vi "PH_Sixpack_Switch.ProcCases.vi"(0 "i ref in":refnum<vi>, 1 "selector":string, 2 "Data":T1, 3 "call cluster":T2={"Object"="", "Selector"="", "CallType"=enum."synchronous", "Async Object"="", "Async Selector"="", "Data Descriptor"="", "Data"=[], "Error #"=0, "Expire"=0}, 5 "error in (no error)":errorcluster) -> (14 "i ref out":refnum<vi>, 17 "answer cluster":T2={"Object"="", "Selector"="", "CallType"=enum."synchronous", "Async Object"="", "Async Selector"="", "Data Descriptor"="", "Data"=[], "Error #"=0, "Expire"=0}, 19 "error out":errorcluster)   [LabVIEW 2014, in "PH_Sixpack_Switch.lvlib"]
doc: "This method is called by a process from within the default case in the event loop. The methods of a class that are linked to events will be called from THIS method. Add your code here."
uses:
  PH_Sixpack_Switch.lvlib
  CS_Core/CSSystem/CoreDefs/CoreDefs.call_type.ctl
  CS_Core/BaseProcess/BaseProcess.descriptor string definition.ctl
  CS_Core/CSSystem/CoreDefs/CoreDefs.rawDataType.ctl
  CS_Core/CSSystem/CoreLib/CoreLib.string 2 byte array.vi
  CS_Core/CSSystem/CoreLib/CoreLib.byte array 2 short.vi
  CS_Core/CSSystem/CoreLib/CoreLib.lvlib
  CS_Core/BaseProcess/BaseProcess.lvlib
  CS_Core/CAEObj/CAEObj.lvlib
  PH_Basics/PH_PSDBWriter/PH_PSDBWriter.lvlib
  PH_Basics/PH_AxisGUI_BaseClass/PH_AxisGUI_BaseClass.lvlib
  PH_Basics/PH_Stepmotor_BaseClass/PH_Stepmotor_BaseClass.lvlib
  PH_AxisGUI_6P/PH_AxisGUI_6P.lvlib
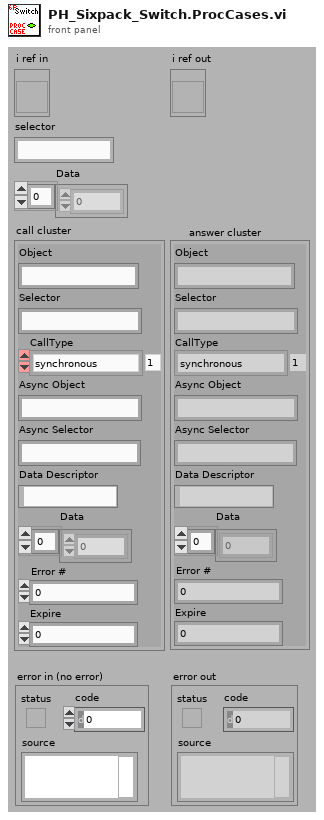
[diagram p1: front panel]
types:
  T1 = typedef "CoreDefs.rawDataType.ctl" = i8[]
  T2 = typedef "CoreDefs.call_type.ctl" = cluster{"Object":string, "Selector":string, "CallType":enum16{"simple", "synchronous", "asynchronous"}, "Async Object":string, "Async Selector":string, "Data Descriptor":T3, "Data":T1, "Error #":i32, "Expire":u32}
  T3 = typedef "BaseProcess.lvlib/BaseProcess.descriptor string definition.ctl" = string
  T4 = enum8{"Enabled", "Disabled", "Disabled and Grayed Out"}
  T5 = typedef "PH_Sixpack_Switch.lvlib/PH_Sixpack_Switch.i attribute.ctl" = cluster{"GUI Refs":cluster{"Delete":refnum<vi>, "Move":refnum<vi>, "Direction":refnum<vi>}, "remote controlled?":bool, "Move":bool, "Direction":T6}
  T6 = typedef "PH_Stepmotor_BaseClass.lvlib/PH_Stepmotor_BaseClass.Axis Direction.ctl" = enum16{"forward", "backward"}
  T7 = typedef "PH_Stepmotor_BaseClass.lvlib/PH_Stepmotor_BaseClass.Axis Information.ctl" = cluster{"Scaled Position":dbl, "Activity":T8}
  T8 = typedef "PH_Stepmotor_BaseClass.lvlib/PH_Stepmotor_BaseClass.Axis Activity.ctl" = enum16{"No Information", "stopped", "running", "Failure", "Alarm", "stopped at backward ES", "stopped at foreward ES"}
  T9 = typedef "PH_AxisGUI_BaseClass.lvlib/PH_AxisGUI_BaseClass.i attribute.ctl" = cluster{"Axes":T10[]}
  T10 = typedef "PH_AxisGUI_BaseClass.lvlib/PH_AxisGUI_BaseClass.Axis Attributes.ctl" = cluster{"Axis GUI Refs":T11, "Address":T12, "Name":string, "Label \"Back\"":string, "Labell \"Forth\"":string, "Moving?":bool}
  T11 = typedef "PH_AxisGUI_BaseClass.lvlib/PH_AxisGUI_BaseClass.Axis GUI Refs.ctl" = cluster{"Back":refnum<vi>, "Forth":refnum<vi>, "Status":refnum<vi>, "Target":refnum<vi>, "Address":refnum<vi>, "Status Bar":refnum<vi>, "Settings":refnum<vi>, "Activity":refnum<vi>, "Clear Error":refnum<vi>}
  T12 = typedef "PH_Stepmotor_BaseClass.lvlib/PH_Stepmotor_BaseClass.Axis Address.ctl" = cluster{"Instance":string, "Motor Nr":i32}
  T13 = typedef "PH_PSDBWriter.lvlib/PH_PSDBWriter.PHELIX-Subsystems.ctl" = i32
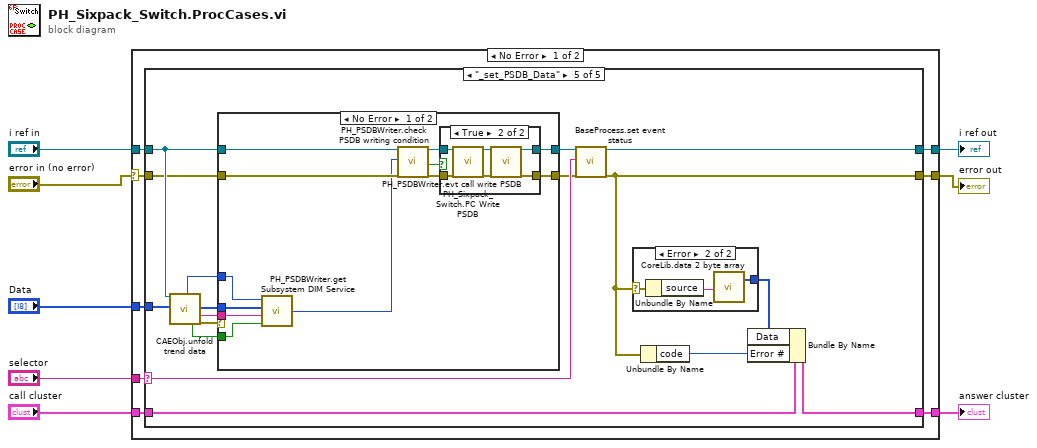
[diagram p0: block diagram]
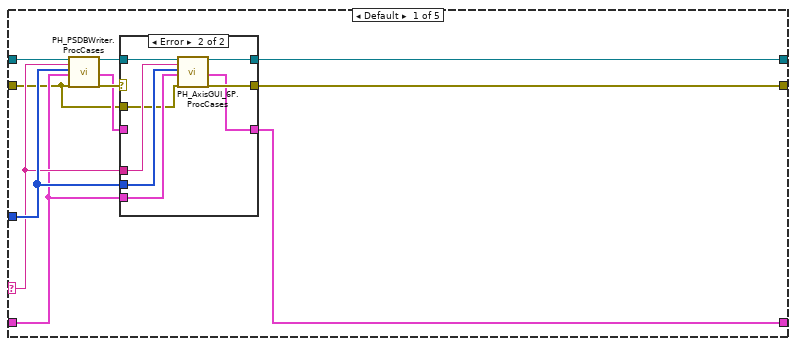
[diagram p2: hidden frame]
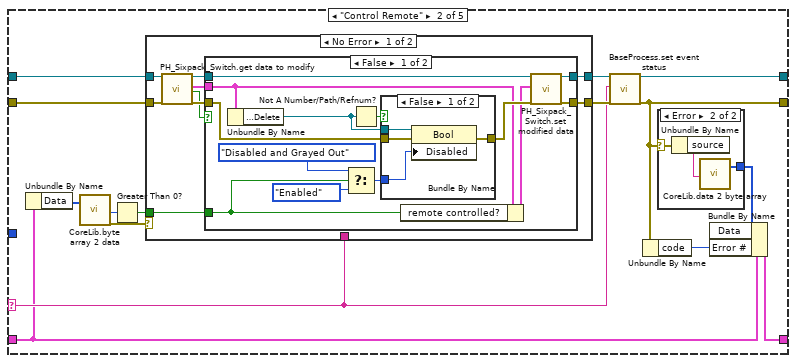
[diagram p4: hidden frame]
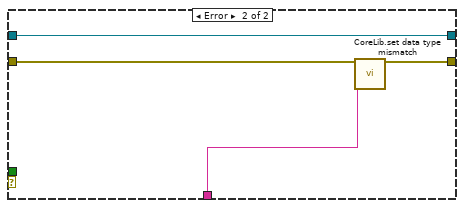
[diagram p8: hidden frame]
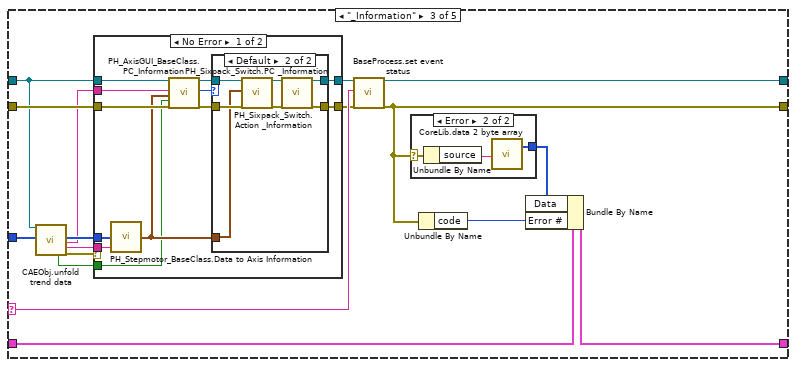
[diagram p9: hidden frame]
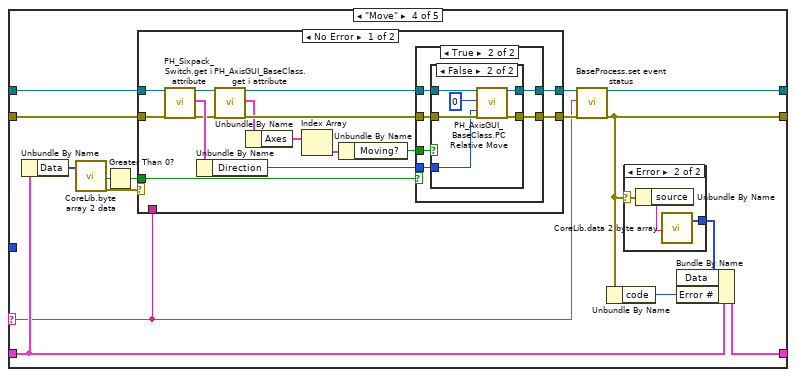
[diagram p13: hidden frame]
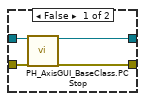
[diagram p14: hidden frame]
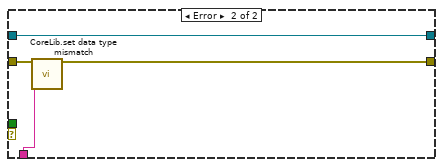
[diagram p16: hidden frame]
diagram:
  n1 = case shown="No Error" "error in (no error)" {
    selector: "error in (no error)" -> [w9 w231]
    tunnel: "selector" -> [w16 _]
    tunnel: [w15 w230] -> w7
    tunnel: "call cluster" -> [w14 w230]
    tunnel: "i ref in" -> [w13 w232]
    tunnel: [w12 w232] -> w4
    tunnel: [w11 w231] -> w3
    tunnel: "Data" -> [w10 _]
    frame No Error {
      n2 = case shown="\"_set_PSDB_Data\"" w16 {
        selector: w16 -> [w19 w41 w102 w134 w198]
        tunnel: w13 -> [w26 w45 w91 w139 w192]
        tunnel: [w25 w43 w104 w145 w202] -> w12
        tunnel: w14 -> [w18 w40 w101 w137 w199]
        tunnel: [w21 w39 w100 w143 w200] -> w15
        tunnel: w9 -> [w17 w44 w94 w141 w191]
        tunnel: [w24 w42 w103 w144 w201] -> w11
        tunnel: w10 -> [w20 _ w99 _ w190]
        frame Default {
          n3 = call "PH_PSDBWriter.ProcCases.vi"("i ref in"=w26, "selector"=w19, "Data"=w20, "call cluster"=w18, "error in"=w17) -> ("i ref out"=w27:refnum<vi>, "answer cluster"=w22:T2, "error out"=w23:errorcluster)  [unwired: 12 in]
          n4 = case shown="Error" w23 {
            selector: w23 -> [w29 _]
            tunnel: w27 -> [w30 w38]
            tunnel: [w30 w37] -> w25
            tunnel: [w29 w36] -> w24
            tunnel: w22 -> [w28 _]
            tunnel: [w28 w35] -> w21
            tunnel: w20 -> [_ w34]
            tunnel: w19 -> [_ w33]
            tunnel: w18 -> [_ w32]
            tunnel: w17 -> [_ w31]
            frame No Error {
            }
            frame Error {
              n5 = call "PH_AxisGUI_6P.ProcCases.vi"("i ref in"=w38, "selector"=w33, "data"=w34, "call cluster"=w32, "error in"=w31) -> ("i ref out"=w37:refnum<vi>, "answer cluster"=w35:T2, "error out"=w36:errorcluster)  [unwired: 12 in]
            }
          }
        }
        frame "Control Remote" {
          n6 = Unbundle By Name(w40) -> ("Data"=w48:T1)
          n7 = call-poly "CoreLib.byte array 2 data.vi"("byteArray"=w48) -> ("i16"=w49:i16, "error out"=w51:errorcluster)  [unwired: 16 in, 1 out]
          n8 = Greater Than 0?(x=w49) -> (x > 0?=w50:bool)
          n9 = case shown="No Error" w51 {
            tunnel: [w58 w89] -> w46
            tunnel: w45 -> [w65 w89]
            tunnel: w44 -> [w64 w88]
            tunnel: [w60 w87] -> w47
            tunnel: w41 -> [_ w86]
            tunnel: w50 -> [w62 _]
            frame No Error {
              n10 = call "PH_Sixpack_Switch.get data to modify.vi"("i ref in"=w65, "error in (no error)"=w64) -> ("i ref out"=w59:refnum<vi>, "i attribute"=w63:T5, "timed out"=w57:bool, "error out"=w61:errorcluster)  [unwired: 14 in]
              n11 = case shown="False" w57 {
                tunnel: w63 -> [w73 _]
                tunnel: w62 -> [w71 _]
                tunnel: w61 -> [w78 w84]
                tunnel: [w77 w84] -> w60
                tunnel: w59 -> [w75 w85]
                tunnel: [w74 w85] -> w58
                frame False {
                  n12 = Unbundle By Name(w73) -> ("GUI Refs.Delete"=w69:refnum<vi>)
                  n13 = Select(t=T4."Disabled and Grayed Out", s=w71, f=T4."Enabled" ("Disabled")) -> (s? t:f=w70:T4)
                  n14 = Not A Number/Path/Refnum?(number/path/refnum=w69) -> (NaN/Path/Refnum?=w68:bool)
                  n15 = case shown="False" w68 {
                    tunnel: w69 -> [w82 _]
                    tunnel: w78 -> [w81 w83]
                    tunnel: [w80 w83] -> w76
                    tunnel: w70 -> [w79 _]
                    frame False {
                      n16 = property class="Bool"(reference=w82, error in=w81, "Disabled"=w79) -> (error out=w80:errorcluster)  [unwired: 1 out]
                    }
                    frame True {
                    }
                  }
                  n17 = Bundle By Name(cluster=w73, "remote controlled?"=w71) -> (w72:T5)
                  n18 = call "PH_Sixpack_Switch.set modified data.vi"("i ref in"=w75, "i attribute"=w72, "error in (no error)"=w76) -> ("i ref out"=w74:refnum<vi>, "error out"=w77:errorcluster)  [unwired: 15 in]
                }
                frame True {
                }
              }
            }
            frame Error {
              n19 = call "CoreLib.set data type mismatch.vi"("error in (no error)"=w88, "error source"=w86) -> ("error out"=w87:errorcluster)  [unwired: 17 in]
            }
          }
          n20 = call "BaseProcess.set event status.vi"("i ref in"=w46, "EventStatus"=w41, "error in (no error)"=w47) -> ("i ref out"=w43:refnum<vi>, "error out"=w42:errorcluster)  [unwired: 14 in, 1 out]
          n21 = Unbundle By Name(w42) -> ("code"=w52:i32)
          n22 = case shown="Error" w42 {
            selector: w42 -> [_ w56]
            tunnel: [_ w54] -> w53
            frame No Error {
            }
            frame Error {
              n23 = Unbundle By Name(w56) -> ("source"=w55:string)
              n24 = call-poly "CoreLib.data 2 byte array.vi"("string"=w55) -> ("byteArray out"=w54:T1)  [unwired: 18 in]
            }
          }
          n25 = Bundle By Name(cluster=w40, "Data"=w53, "Error #"=w52) -> (w39:T2)
        }
        frame "_Information" {
          n26 = call "CAEObj.unfold trend data.vi"("i ref in"=w91, "raw trend data"=w99) -> ("no link"=w92:bool, "data"=w98:i8[], "serviceName"=w90:string, "typeDescriptor"=w97:string, "error out"=w96:errorcluster)  [unwired: 9 in, 4 out]
          n27 = case shown="No Error" w96 {
            tunnel: w98 -> [w111 _]
            tunnel: w97 -> [w110 _]
            tunnel: w91 -> [w114 w129]
            tunnel: [w117 w129] -> w95
            tunnel: w94 -> [w118 w128]
            tunnel: [w116 w128] -> w93
            tunnel: w92 -> [w107 _]
            tunnel: w90 -> [w112 _]
            frame No Error {
              n28 = call "PH_Stepmotor_BaseClass.Data to Axis Information.vi"("data"=w111, "Type Descriptor"=w110) -> ("Axis Information"=w108:T7)
              n29 = call "PH_AxisGUI_BaseClass.PC_Information.vi"("i ref in"=w114, "Service Name"=w112, "Axis Information"=w108, "no link"=w107, "error in"=w118) -> ("i ref out"=w113:refnum<vi>, "Axis"=w109:i32, "error out"=w115:errorcluster)  [unwired: 12 in]
              n30 = case shown="Default" w109 {
                tunnel: [w120 w122] -> w117
                tunnel: [w119 w121] -> w116
                tunnel: w115 -> [w119 w125]
                tunnel: w113 -> [w120 w124]
                tunnel: w108 -> [_ w123]
                frame -1 {
                }
                frame Default {
                  n31 = call "PH_Sixpack_Switch.PC _Information.vi"("i ref in"=w124, "Axis Information"=w123, "error IO"=w125) -> ("i ref out"=w127:refnum<vi>, "error out"=w126:errorcluster)  [unwired: 15 in]
                  n32 = call "PH_Sixpack_Switch.Action _Information.vi"("i ref in"=w127, "error IO"=w126) -> ("i ref out"=w122:refnum<vi>, "error out"=w121:errorcluster)  [unwired: 16 in]
                }
              }
            }
            frame Error {
            }
          }
          n33 = call "BaseProcess.set event status.vi"("i ref in"=w95, "EventStatus"=w102, "error in (no error)"=w93) -> ("i ref out"=w104:refnum<vi>, "error out"=w103:errorcluster)  [unwired: 14 in, 1 out]
          n34 = case shown="Error" w103 {
            selector: w103 -> [_ w132]
            tunnel: [_ w130] -> w106
            frame No Error {
            }
            frame Error {
              n35 = Unbundle By Name(w132) -> ("source"=w131:string)
              n36 = call-poly "CoreLib.data 2 byte array.vi"("string"=w131) -> ("byteArray out"=w130:T1)  [unwired: 18 in]
            }
          }
          n37 = Unbundle By Name(w103) -> ("code"=w105:i32)
          n38 = Bundle By Name(cluster=w101, "Data"=w106, "Error #"=w105) -> (w100:T2)
        }
        frame "Move" {
          n39 = Unbundle By Name(w137) -> ("Data"=w138:T1)
          n40 = call-poly "CoreLib.byte array 2 data.vi"("byteArray"=w138) -> ("i16"=w135:i16, "error out"=w136:errorcluster)  [unwired: 16 in, 1 out]
          n41 = Greater Than 0?(x=w135) -> (x > 0?=w133:bool)
          n42 = case shown="No Error" w136 {
            tunnel: w139 -> [w162 w184]
            tunnel: [w159 w184] -> w142
            tunnel: w141 -> [w161 w183]
            tunnel: [w158 w182] -> w140
            tunnel: w134 -> [_ w181]
            tunnel: w133 -> [w160 _]
            frame No Error {
              n43 = call "PH_Sixpack_Switch.get i attribute.vi"("i ref in"=w162, "error in (no error)"=w161) -> ("i ref out"=w154:refnum<vi>, "i attribute"=w157:T5, "error out"=w156:errorcluster)  [unwired: 15 in]
              n44 = Unbundle By Name(w157) -> ("Direction"=w148:T6)
              n45 = call "PH_AxisGUI_BaseClass.get i attribute.vi"("i ref in"=w154, "error in (no error)"=w156) -> ("i ref out"=w153:refnum<vi>, "i attribute"=w152:T9, "error out"=w155:errorcluster)  [unwired: 15 in]
              n46 = Unbundle By Name(w152) -> ("Axes"=w151:T10[])
              n47 = Index Array(array=w151) -> (element=w150:T10)  [unwired: 1 in]
              n48 = Unbundle By Name(w150) -> ("Moving?"=w149:bool)
              n49 = case shown="True" w160 {
                tunnel: w153 -> [w166 w172]
                tunnel: w155 -> [w165 w170]
                tunnel: [w164 w169] -> w158
                tunnel: [w163 w171] -> w159
                tunnel: w149 -> [_ w168]
                tunnel: w148 -> [_ w167]
                frame False {
                  n50 = call "PH_AxisGUI_BaseClass.PC Stop.vi"("VI in"=w166, "error in (no error)"=w165) -> ("VI out"=w163:refnum<vi>, "error out"=w164:errorcluster)  [unwired: 16 in]
                }
                frame True {
                  n51 = case shown="False" w168 {
                    tunnel: w172 -> [w174 w180]
                    tunnel: [w174 w179] -> w171
                    tunnel: w170 -> [w173 w178]
                    tunnel: [w173 w177] -> w169
                    tunnel: w167 -> [_ w176]
                    frame True {
                    }
                    frame False {
                      n52 = call "PH_AxisGUI_BaseClass.PC Relative Move.vi"("i ref in"=w180, "Axis"=0, "direction"=w176, "error in"=w178) -> ("i ref out"=w179:refnum<vi>, "error out"=w177:errorcluster)  [unwired: 14 in]
                    }
                  }
                }
              }
            }
            frame Error {
              n53 = call "CoreLib.set data type mismatch.vi"("error in (no error)"=w183, "error source"=w181) -> ("error out"=w182:errorcluster)  [unwired: 17 in]
            }
          }
          n54 = call "BaseProcess.set event status.vi"("i ref in"=w142, "EventStatus"=w134, "error in (no error)"=w140) -> ("i ref out"=w145:refnum<vi>, "error out"=w144:errorcluster)  [unwired: 14 in, 1 out]
          n55 = Unbundle By Name(w144) -> ("code"=w146:i32)
          n56 = case shown="Error" w144 {
            selector: w144 -> [_ w187]
            tunnel: [_ w185] -> w147
            frame No Error {
            }
            frame Error {
              n57 = Unbundle By Name(w187) -> ("source"=w186:string)
              n58 = call-poly "CoreLib.data 2 byte array.vi"("string"=w186) -> ("byteArray out"=w185:T1)  [unwired: 18 in]
            }
          }
          n59 = Bundle By Name(cluster=w137, "Data"=w147, "Error #"=w146) -> (w143:T2)
        }
        frame "_set_PSDB_Data" {
          n60 = call "CAEObj.unfold trend data.vi"("i ref in"=w192, "raw trend data"=w190) -> ("quality"=w193:i32, "no link"=w196:bool, "data"=w194:i8[], "typeDescriptor"=w195:string, "error out"=w197:errorcluster)  [unwired: 9 in, 4 out]
          n61 = case shown="No Error" w197 {
            tunnel: w191 -> [w216 w226]
            tunnel: [w215 w225] -> w189
            tunnel: [w214 w226] -> w188
            tunnel: w192 -> [w212 w225]
            tunnel: w196 -> [w207 _]
            tunnel: w195 -> [w205 _]
            tunnel: w194 -> [w209 _]
            tunnel: w193 -> [w208 _]
            frame No Error {
              n62 = call "PH_PSDBWriter.get Subsystem DIM Service.vi"("no link"=w207, "typeDescriptor"=w205, "data"=w209, "quality"=w208) -> ("PHELIX Subsystems"=w206:T13)
              n63 = call "PH_PSDBWriter.check PSDB writing condition.vi"("i ref in"=w212, "wanted Subsystem"=w206, "error IO"=w216) -> ("i ref out"=w211:refnum<vi>, "write PSDB?"=w210:bool, "error out"=w213:errorcluster)  [unwired: 14 in]
              n64 = case shown="True" w210 {
                tunnel: w213 -> [w217 w224]
                tunnel: [w218 w221] -> w215
                tunnel: [w217 w219] -> w214
                tunnel: w211 -> [w218 w223]
                frame False {
                }
                frame True {
                  n65 = call "PH_Sixpack_Switch.PC Write PSDB.vi"("i ref in"=w223, "error IO"=w224) -> ("i ref out"=w222:refnum<vi>, "error out"=w220:errorcluster)  [unwired: 16 in]
                  n66 = call "PH_PSDBWriter.evt call write PSDB.vi"("i ref in"=w222, "error in (no error)"=w220) -> ("i ref out"=w221:refnum<vi>, "error out"=w219:errorcluster)  [unwired: 16 in]
                }
              }
            }
            frame Error {
            }
          }
          n67 = call "BaseProcess.set event status.vi"("i ref in"=w189, "EventStatus"=w198, "error in (no error)"=w188) -> ("i ref out"=w202:refnum<vi>, "error out"=w201:errorcluster)  [unwired: 14 in, 1 out]
          n68 = case shown="Error" w201 {
            selector: w201 -> [_ w229]
            tunnel: [_ w227] -> w204
            frame No Error {
            }
            frame Error {
              n69 = Unbundle By Name(w229) -> ("source"=w228:string)
              n70 = call-poly "CoreLib.data 2 byte array.vi"("string"=w228) -> ("byteArray out"=w227:T1)  [unwired: 18 in]
            }
          }
          n71 = Unbundle By Name(w201) -> ("code"=w203:i32)
          n72 = Bundle By Name(cluster=w199, "Data"=w204, "Error #"=w203) -> (w200:T2)
        }
      }
    }
    frame Error {
    }
  }
  "answer cluster" <- w7
  "i ref out" <- w4
  "error out" <- w3
